vi "ErrorCountUpdated.vi"(8 "error in (no error)":errorcluster, 10 "ErrorCount":u32, 11 "TCP_Client in":refnum<class "TCP_Client.lvclass">) -> (0 "error out":errorcluster, 3 "TCP_Client out":refnum<class "TCP_Client.lvclass">)   [LabVIEW 2023, in "TCP_Client.lvlib" / "TCP_Client.lvclass"]
uses:
  TCP_Client.lvclass
  TCP_Client.lvclass/TCP_Client.ctl
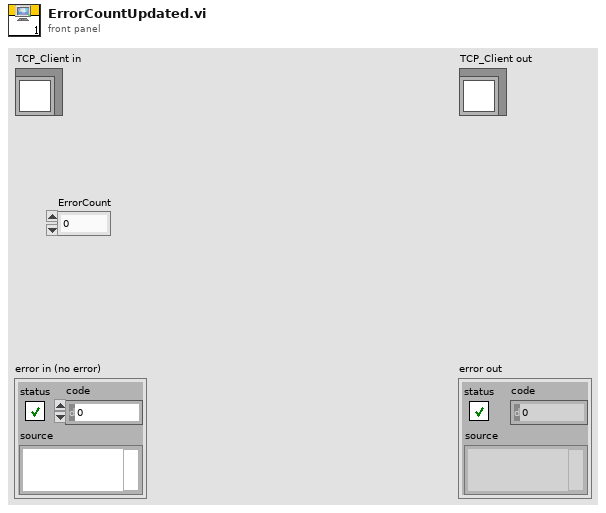
[diagram p1: front panel]
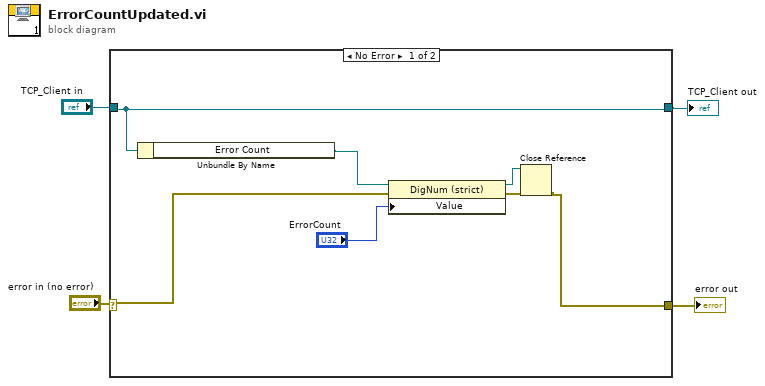
[diagram p0: block diagram]
diagram:
  n1 = case shown="No Error" "error in (no error)" {
    selector: "error in (no error)" -> [w9 w13]
    tunnel: [w6 w13] -> w3
    tunnel: "TCP_Client in" -> [w5 w12]
    tunnel: [w5 w12] -> w1
    frame No Error {
      n2 = Unbundle By Name(w5) -> ("Error Count"=w11:refnum<vi>)
      n3 = property class="DigNum (strict)"(reference=w11, error in=w9, "Value"="ErrorCount") -> (reference out=w7:refnum<vi>, error out=w8:errorcluster)
      n4 = Close Reference(reference=w7, error in (no error)=w8) -> (error out=w6:errorcluster)
    }
    frame Error {
    }
  }
  "error out" <- w3
  "TCP_Client out" <- w1
